vi "XYZ Step.vi"(1 "Step Size":dbl, 2 "Negative":bool, 3 "Positive":bool) -> (0 "Relative Movement":dbl)   [LabVIEW 2014]
panel:
  # "LICENSED MATERIALS – PROPERTY OF IBM\nCopyright IBM Corp. 2016,\nALL RIGHTS RESERVED"
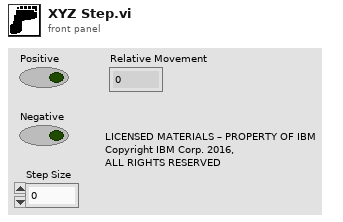
[diagram p1: front panel]
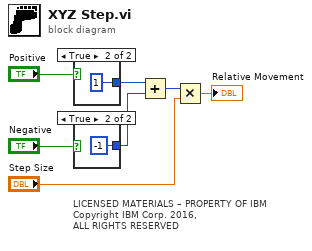
[diagram p0: block diagram]
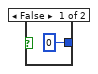
[diagram p2: hidden frame]
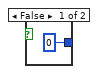
[diagram p3: hidden frame]
diagram:
  # "LICENSED MATERIALS – PROPERTY OF IBM\nCopyright IBM Corp. 2016,\nALL RIGHTS RESERVED"
  n1 = case shown="True" "Positive" {
    tunnel: [0 1] -> w2
    frame False {
    }
    frame True {
    }
  }
  n2 = case shown="True" "Negative" {
    tunnel: [0 -1] -> w4
    frame False {
    }
    frame True {
    }
  }
  n3 = Add(x=w2, y=w4) -> (x+y=w5:i32)
  n4 = Multiply(x=w5, y="Step Size") -> (x*y=→"Relative Movement":dbl)
